vi "DAC.vi"(8 "error in (no error)":errorcluster, 9 "DAC":u8(knob) scale=0.0..255.0, 10 "Pin":u8=25 min=25 max=26, 11 "VISA resource name":refnum<visa-resource-name>) -> (0 "error out":errorcluster, 2 "Voltaje":dbl, 3 "VISA resource name out":refnum<visa-resource-name>)   [LabVIEW 2025]
doc: "Este VI permite usar el DAC de 8 bits que tienen las ESP32, este solo se limita a algunos pines para garantizar su uso \nSe debe ingresar el valor del DAC deseado NO el voltaje \nEl DAC es capaz de suministrar de 0 a 3.3V"
panel:
  out "read buffer":string
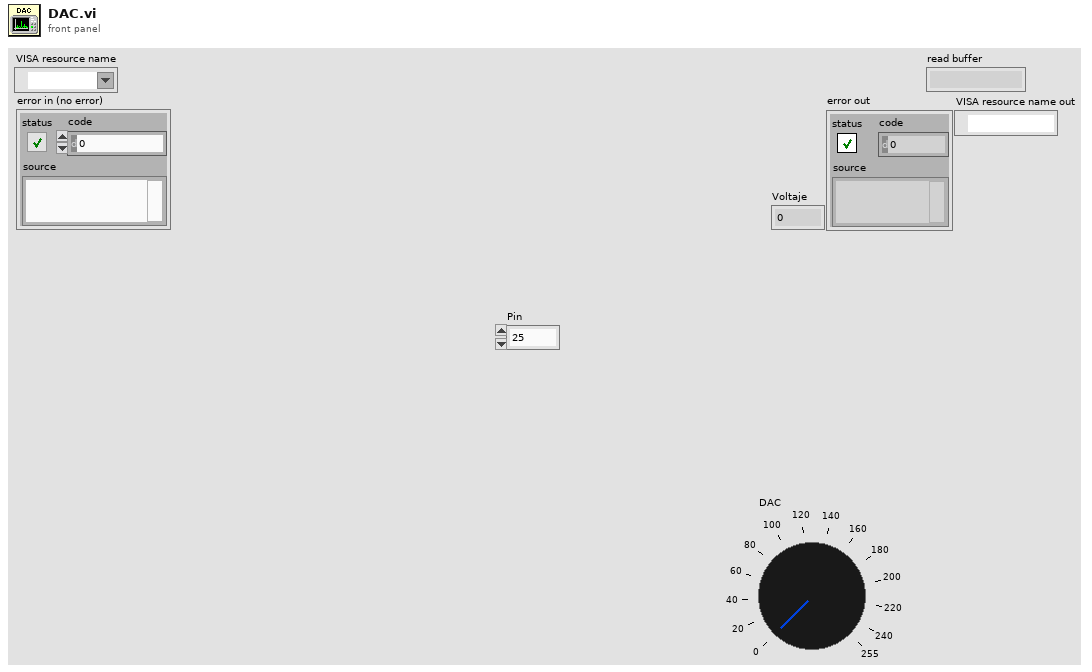
[diagram p1: front panel]
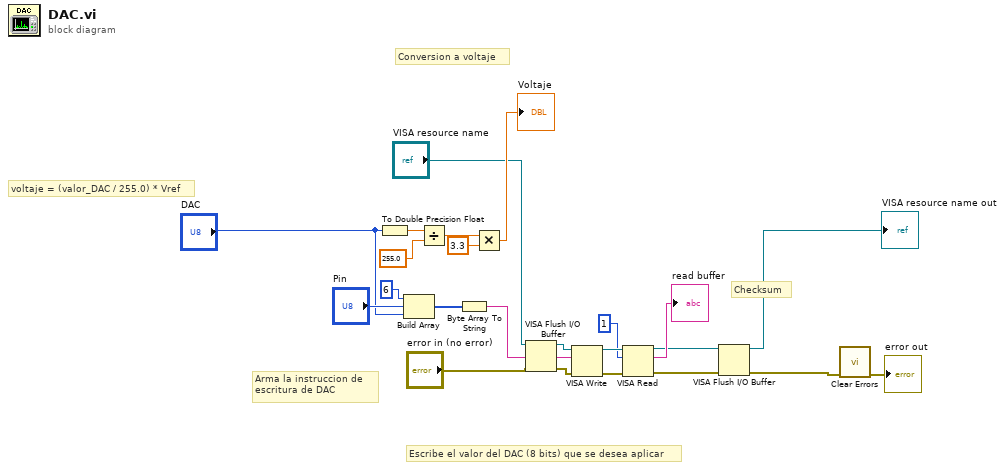
[diagram p0: block diagram]
diagram:
  # "Checksum"
  # "Conversion a voltaje"
  # "Escribe el valor del DAC (8 bits) que se desea aplicar"
  # "Arma la instruccion de \nescritura de DAC"
  # "voltaje = (valor_DAC / 255.0) * Vref"
  n1 = To Double Precision Float(number="DAC") -> (double precision float=w9:dbl)
  n2 = Build Array(u8 6, "Pin", "DAC") -> (w20:u8[])
  n3 = Divide(x=w9, y=255.0) -> (x/y=w12:dbl)
  n4 = Byte Array To String(unsigned byte array=w20) -> (string=w23:string)
  n5 = Multiply(x=w12, y=3.3) -> (x*y=→"Voltaje":dbl)
  n6 = VISA Flush I/O Buffer(VISA resource name="VISA resource name", error in (no error)="error in (no error)") -> (VISA resource name out=w1:refnum<visa-resource-name>, error out=w4:errorcluster)  [unwired: 1 in]
  n7 = VISA Write(VISA resource name=w1, write buffer=w23, error in (no error)=w4) -> (VISA resource name out=w19:refnum<visa-resource-name>, error out=w18:errorcluster)  [unwired: 1 out]
  n8 = VISA Read(VISA resource name=w19, byte count=u32 1, error in (no error)=w18) -> (VISA resource name out=w5:refnum<visa-resource-name>, read buffer=→"read buffer":string, error out=w8:errorcluster)  [unwired: 1 out]
  n9 = VISA Flush I/O Buffer(VISA resource name=w5, error in (no error)=w8) -> (VISA resource name out=→"VISA resource name out":refnum<visa-resource-name>, error out=w7:errorcluster)  [unwired: 1 in]
  n10 = call <vilib>:"Clear Errors.vi"("error in (no error)"=w7) -> ("error out"=→"error out":errorcluster)  [unwired: 5 in, 1 out]
